vi "Disconnect.vi"(8 "error in":errorcluster, 11 "6512 in":refnum<class "6512.lvclass">) -> (0 "error out":errorcluster, 3 "6512 out":refnum<class "6512.lvclass">)   [LabVIEW 2019, in "6512.lvlib" / "6512.lvclass"]
uses:
  Library/6512.lvclass
  Library/6512.lvclass/6512.ctl
  Accessors/Read Local Resource.vi
  Accessors/Write Local Resource.vi
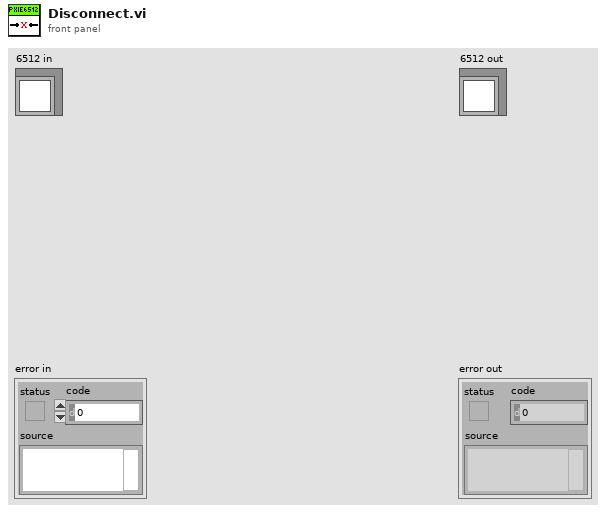
[diagram p1: front panel]
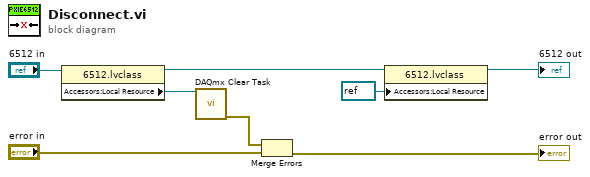
[diagram p0: block diagram]
diagram:
  n1 = property class="6512.lvclass"(reference="6512 in") -> (reference out=w3:refnum<class "6512.lvclass">, "Accessors:Local Resource"=w4:refnum<k21>)  [unwired: 1 in, 1 out]
  n2 = call <vilib>:"DAQmx Clear Task.vi"("task in"=w4) -> ("error out"=w1:errorcluster)  [unwired: 14 in]
  n3 = Merge Errors(w1, "error in") -> (→"error out":errorcluster)
  n4 = property class="6512.lvclass"(reference=w3, "Accessors:Local Resource"=refnum<k21> refnum ("Local Resource")) -> (reference out=→"6512 out":refnum<class "6512.lvclass">)  [unwired: 1 in, 1 out]
